vi "Execute.vi"(8 "error in (no error)":errorcluster, 10 "Motor in":refnum<class "Motor.lvclass">, 11 "Move-timer in":refnum<class "Move-Timer.lvclass">) -> (0 "error out":errorcluster, 1 "Status message":string, 2 "Motor out":refnum<class "Motor.lvclass">, 3 "Move-timer out":refnum<class "Move-Timer.lvclass">)   [LabVIEW 2013, in "PowderDeposition.lvlib" / "Move-Timer.lvclass"]
uses:
  Move-Timer.lvclass
  Motor/Motor.lvclass
  Move-Timer.lvclass/Move-Timer.ctl
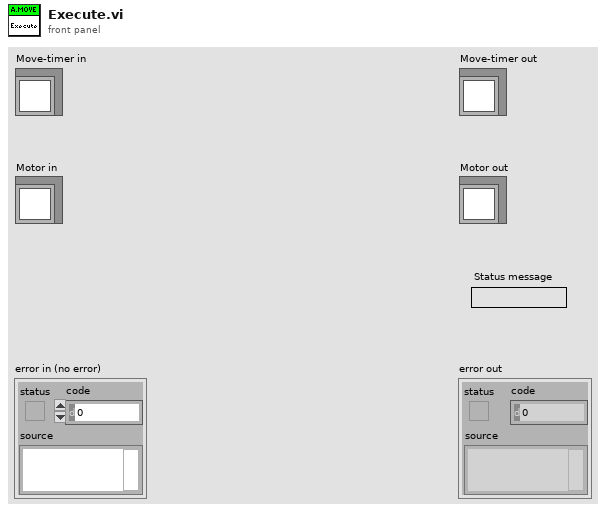
[diagram p1: front panel]
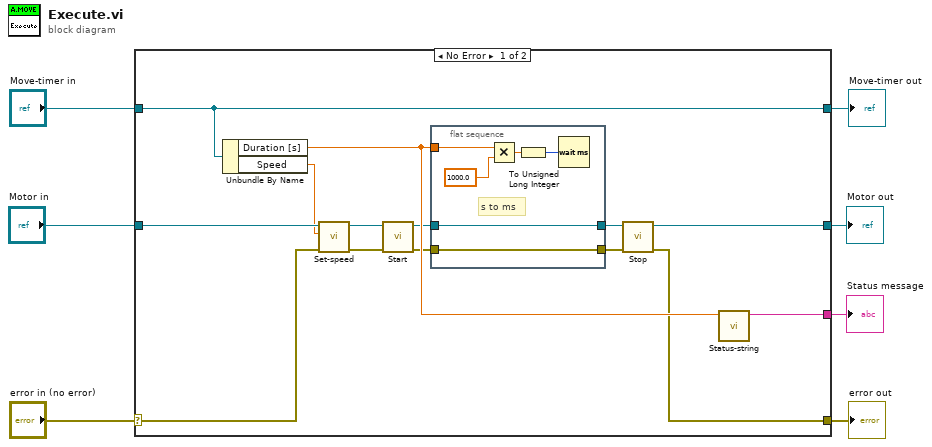
[diagram p0: block diagram]
diagram:
  n1 = case shown="No Error" "error in (no error)" {
    selector: "error in (no error)" -> [w12 w30]
    tunnel: [w8 w30] -> w6
    tunnel: [w21 w29] -> w4
    tunnel: "Move-timer in" -> [w21 w29]
    tunnel: [w19 _] -> w3
    tunnel: "Motor in" -> [w18 w28]
    tunnel: [w11 w28] -> w1
    frame No Error {
      n2 = Unbundle By Name(w21) -> ("Duration [s]"=w20:dbl, "Speed"=w16:dbl)
      n3 = call-dynamic "Set-speed.vi"("error in (no error)"=w12, "Speed"=w16, "Motor in"=w18) -> ("error out"=w13:errorcluster, "Motor out"=w17:refnum<class "Motor.lvclass">)  [unwired: 7 in]
      n4 = call-dynamic "Start.vi"("error in (no error)"=w13, "Motor in"=w17) -> ("error out"=w14:errorcluster, "Motor out"=w15:refnum<class "Motor.lvclass">)  [unwired: 8 in]
      n5 = flat-sequence {
        tunnel: w20 -> [w24]
        tunnel: w15 -> [w23]
        tunnel: w14 -> [w22]
        tunnel: [w23] -> w10
        tunnel: [w22] -> w9
        frame #0 {
          # "s to ms"
          n6 = Multiply(x=w24, y=1000.0) -> (x*y=w27:dbl)
          n7 = To Unsigned Long Integer(number=w27) -> (unsigned 32bit integer=w25:u32)
          n8 = Wait (ms)(milliseconds to wait=w25) -> ()  [unwired: 1 out]
        }
      }
      n9 = call-dynamic "Stop.vi"("error in (no error)"=w9, "Motor in"=w10) -> ("error out"=w8:errorcluster, "Motor out"=w11:refnum<class "Motor.lvclass">)  [unwired: 8 in]
      n10 = call "Status-string.vi"("Duration [s]"=w20) -> ("String"=w19:string)  [unwired: 10 in]
    }
    frame Error {
    }
  }
  "error out" <- w6
  "Move-timer out" <- w4
  "Status message" <- w3
  "Motor out" <- w1
